vi "Read Status.vi"(8 "error in (no error)":errorcluster, 11 "CSM-Helper in":refnum<class "CSM-Helper.lvclass">) -> (0 "error out":errorcluster, 2 "Array 3":cluster{"Status":string, "InState":string}[](array[cluster]), 3 "CSM-Helper out":refnum<class "CSM-Helper.lvclass">)   [LabVIEW 2017, in "CSM-Helper.lvclass"]
uses:
  CSM-Helper.lvclass
  CSM-Helper.lvclass/CSM-Helper.ctl
  <vilib>/Utility/traverseref.llb/TRef TravTarget.ctl
  <vilib>/Utility/traverseref.llb/VI Scripting - Traverse.lvlib
  Utility/_Support/Terminals.llb/csmHelper-Terminals.lvlib
  _Shared/CSM Shared.lvlib
  Communicable State Machine.lvlib
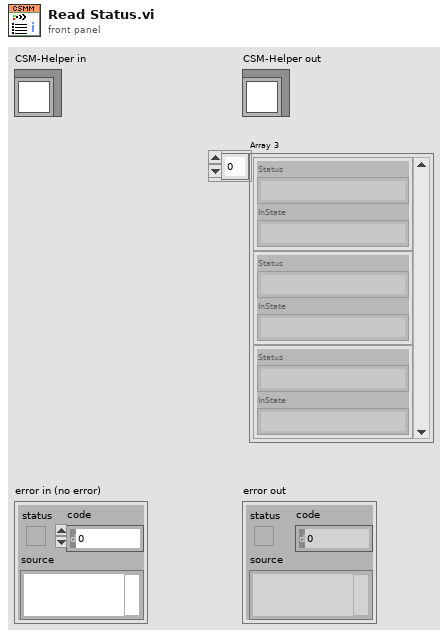
[diagram p1: front panel]
types:
  T1 = typedef "TRef TravTarget.ctl" = enum16{"FP", "BD", "Other"}
  T2 = cluster{"trimed text":string, "trimed text":string}
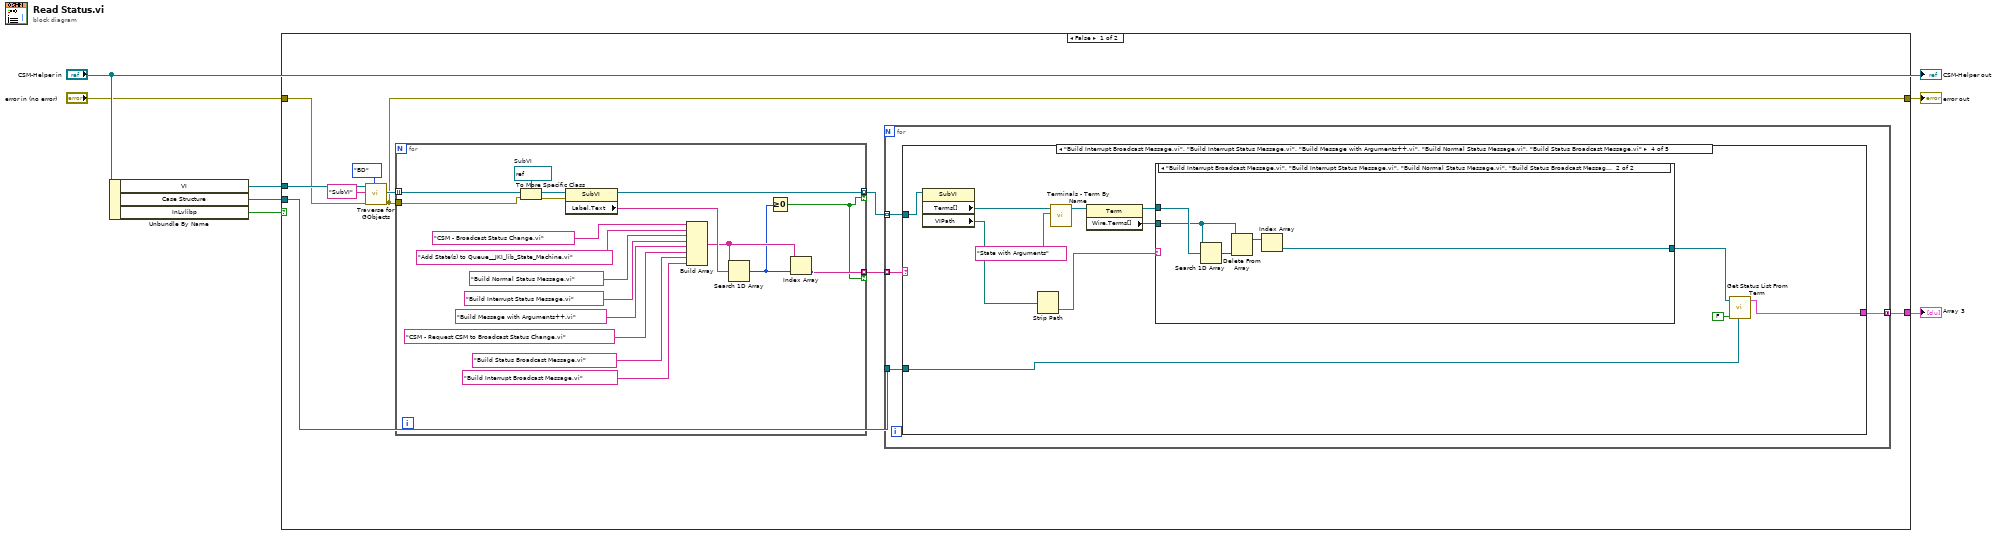
[diagram p0: block diagram]
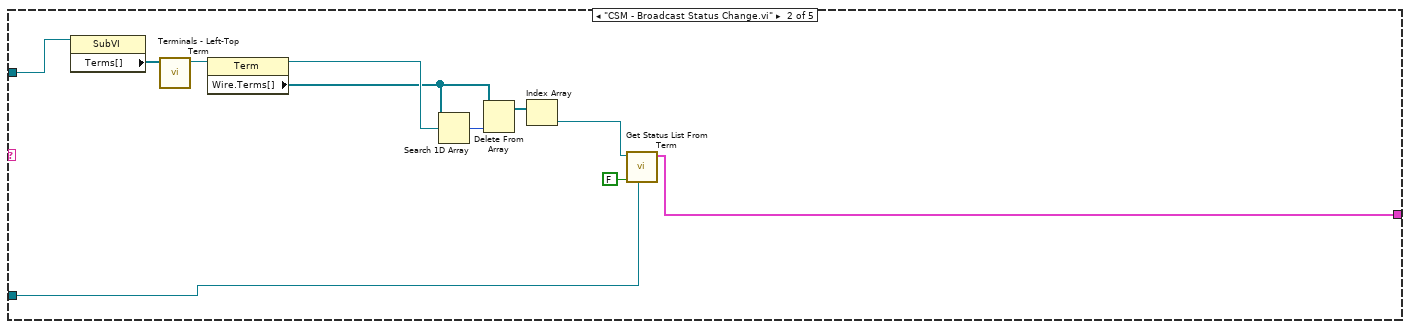
[diagram p3: hidden frame]
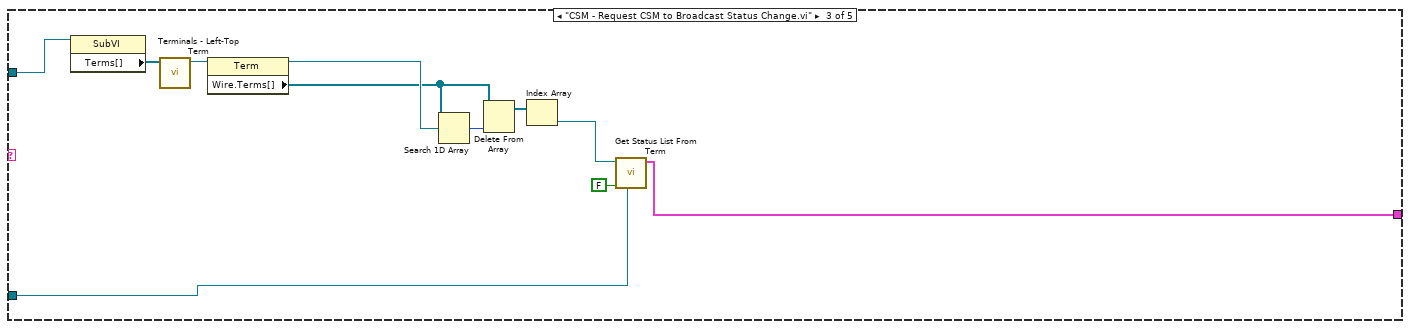
[diagram p4: hidden frame]
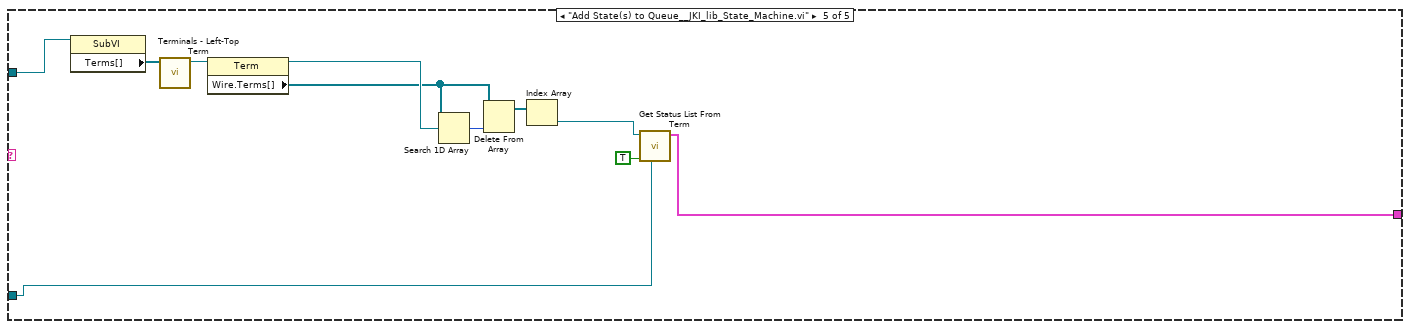
[diagram p6: hidden frame]
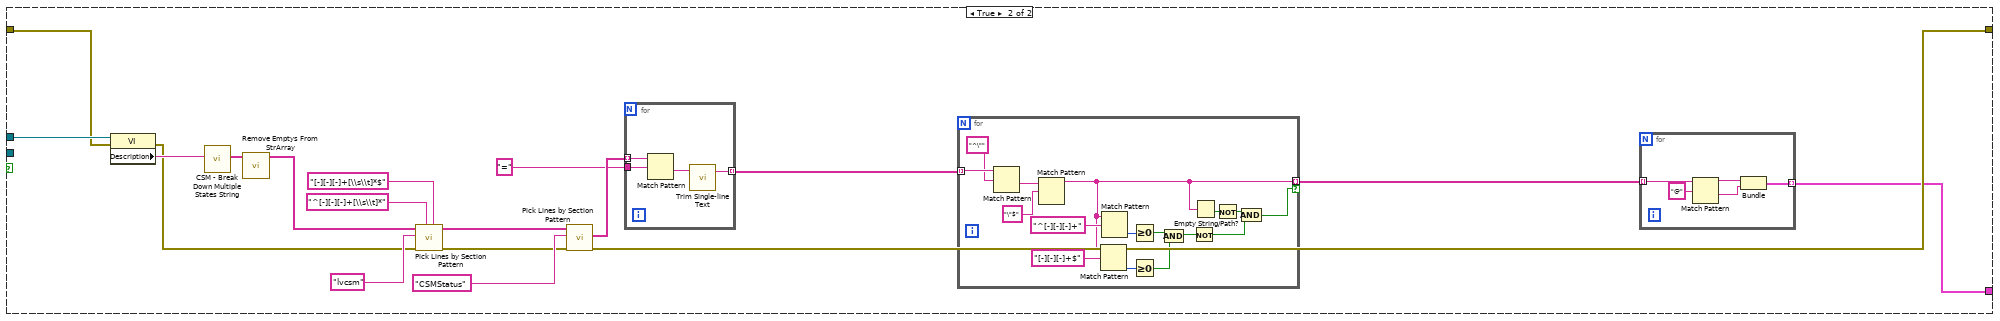
[diagram p7: hidden frame]
diagram:
  n1 = Unbundle By Name("CSM-Helper in") -> ("VI"=w6:refnum<vi>, "Case Structure"=w4:refnum<vi>, "InLvlibp"=w3:bool)
  n2 = case shown="False" w3 {
    tunnel: w6 -> [w13 w96]
    tunnel: [w12 w93] -> w5
    tunnel: w4 -> [w11 _]
    tunnel: "error in (no error)" -> [w9 w95]
    tunnel: [w8 w94] -> w1
    frame False {
      n3 = call <vilib>:"Traverse for GObjects.vi"("Traverse Target"=TRef_TravTarget."BD", "error in (no error)"=w9, "Class Name"="SubVI", "VI Refnum"=w13) -> ("error out"=w8:errorcluster, "References"=w15:refnum<vi>[])  [unwired: 4 in, 2 out]
      n4 = for {
        tunnel: w15 -> [w90] mode=indexing
        tunnel: w8 -> [w86]
        tunnel: [w84] -> w14 mode=indexing if=w78
        tunnel: [w79] -> w10 mode=indexing if=w78
        w87 = refnum<vi> refnum  # SubVI
        n5 = To More Specific Class(target class=w87, reference=w90, error in=w86) -> (specific class reference=w89:refnum<vi>, error out=w88:errorcluster)
        n6 = property class="SubVI"(reference=w89, error in=w88) -> (reference out=w84:refnum<vi>, "Label.Text"=w82:string)  [unwired: 1 out]
        n7 = Build Array("CSM - Broadcast Status Change.vi" ("y"), "Add State(s) to Queue__JKI_lib_State_Machine.vi" ("y"), "Build Normal Status Message.vi" ("y"), "Build Interrupt Status Message.vi" ("y"), "Build Message with Arguments++.vi" ("y"), "CSM - Request CSM to Broadcast Status Change.vi" ("y"), "Build Status Broadcast Message.vi" ("y"), "Build Interrupt Broadcast Message.vi" ("y")) -> (w81:string[])
        n8 = Search 1D Array(1D array=w81, element=w82) -> (index of element=w80:i32)  [unwired: 1 in]
        n9 = Greater Or Equal To 0?(x=w80) -> (x >= 0?=w78:bool)
        n10 = Index Array(array=w81, index=w80) -> (element=w79:string)
      }
      n11 = for {
        tunnel: w14 -> [w21] mode=indexing
        tunnel: [w20] -> w12 mode=concatenating
        tunnel: w11 -> [w19]
        tunnel: w10 -> [w18] mode=indexing
        n12 = case shown="\"Build Interrupt Broadcast Message.vi\", \"Build Interrupt Status Message.vi\", \"Build Message with Arguments++.vi\", \"Build Normal Status Message.vi\", \"Build Status Broadcast Message.vi\"" w18 {
          tunnel: w21 -> [_ w32 w43 w55 w71]
          tunnel: [_ w23 w34 w45 w62] -> w20
          tunnel: w19 -> [_ w24 w35 w47 w63]
          frame Default {
          }
          frame "CSM - Broadcast Status Change.vi" {
            n13 = property class="SubVI"(reference=w32) -> ("Terms[]"=w31:refnum<vi>[])  [unwired: 1 in, 2 out]
            n14 = call "Terminals - Left-Top Term.vi"("Terms[]"=w31) -> ("Terms[] out"=w30:refnum<vi>)  [unwired: 10 in]
            n15 = property class="Term"(reference=w30) -> (reference out=w29:refnum<vi>, "Wire.Terms[]"=w27:refnum<vi>[])  [unwired: 1 in, 1 out]
            n16 = Search 1D Array(1D array=w27, element=w29) -> (index of element=w28:i32)  [unwired: 1 in]
            n17 = Delete From Array(array=w27, index=w28) -> (array with subset deleted=w26:refnum<vi>[])  [unwired: 1 in, 1 out]
            n18 = Index Array(array=w26) -> (element=w25:refnum<vi>)  [unwired: 1 in]
            n19 = call "Get Status List From Term.vi"("CSM CaseRef"=w24, "need Symbol?"=FALSE, "Term Refnum"=w25) -> ("Array"=w23:cluster{"Status":string, "InState":string}[])  [unwired: 6 in]
          }
          frame "CSM - Request CSM to Broadcast Status Change.vi" {
            n20 = property class="SubVI"(reference=w43) -> ("Terms[]"=w42:refnum<vi>[])  [unwired: 1 in, 2 out]
            n21 = call "Terminals - Left-Top Term.vi"("Terms[]"=w42) -> ("Terms[] out"=w41:refnum<vi>)  [unwired: 10 in]
            n22 = property class="Term"(reference=w41) -> (reference out=w40:refnum<vi>, "Wire.Terms[]"=w38:refnum<vi>[])  [unwired: 1 in, 1 out]
            n23 = Search 1D Array(1D array=w38, element=w40) -> (index of element=w39:i32)  [unwired: 1 in]
            n24 = Delete From Array(array=w38, index=w39) -> (array with subset deleted=w37:refnum<vi>[])  [unwired: 1 in, 1 out]
            n25 = Index Array(array=w37) -> (element=w36:refnum<vi>)  [unwired: 1 in]
            n26 = call "Get Status List From Term.vi"("CSM CaseRef"=w35, "need Symbol?"=FALSE, "Term Refnum"=w36) -> ("Array"=w34:cluster{"Status":string, "InState":string}[])  [unwired: 6 in]
          }
          frame "Build Interrupt Broadcast Message.vi", "Build Interrupt Status Message.vi", "Build Message with Arguments++.vi", "Build Normal Status Message.vi", "Build Status Broadcast Message.vi" {
            n27 = property class="SubVI"(reference=w55) -> ("Terms[]"=w52:refnum<vi>[], "VIPath"=w49:path)  [unwired: 1 in, 2 out]
            n28 = Strip Path(path=w49) -> (name=w48:string)  [unwired: 1 out]
            n29 = call "Terminals - Term By Name.vi"("String"="State with Arguments", "Terms[]"=w52) -> ("Terms[] out"=w51:refnum<vi>)  [unwired: 9 in]
            n30 = property class="Term"(reference=w51) -> (reference out=w54:refnum<vi>, "Wire.Terms[]"=w53:refnum<vi>[])  [unwired: 1 in, 1 out]
            n31 = case shown="\"Build Interrupt Broadcast Message.vi\", \"Build Interrupt Status Message.vi\", \"Build Normal Status Message.vi\", \"Build Status Broadcast Message.vi\"" w48 {
              tunnel: w54 -> [_ w60]
              tunnel: w53 -> [_ w58]
              tunnel: [_ w56] -> w46
              frame "False", Default {
              }
              frame "Build Interrupt Broadcast Message.vi", "Build Interrupt Status Message.vi", "Build Normal Status Message.vi", "Build Status Broadcast Message.vi" {
                n32 = Search 1D Array(1D array=w58, element=w60) -> (index of element=w59:i32)  [unwired: 1 in]
                n33 = Delete From Array(array=w58, index=w59) -> (array with subset deleted=w57:refnum<vi>[])  [unwired: 1 in, 1 out]
                n34 = Index Array(array=w57) -> (element=w56:refnum<vi>)  [unwired: 1 in]
              }
            }
            n35 = call "Get Status List From Term.vi"("CSM CaseRef"=w47, "need Symbol?"=FALSE, "Term Refnum"=w46) -> ("Array"=w45:cluster{"Status":string, "InState":string}[])  [unwired: 6 in]
          }
          frame "Add State(s) to Queue__JKI_lib_State_Machine.vi" {
            n36 = property class="SubVI"(reference=w71) -> ("Terms[]"=w70:refnum<vi>[])  [unwired: 1 in, 2 out]
            n37 = call "Terminals - Left-Top Term.vi"("Terms[]"=w70) -> ("Terms[] out"=w69:refnum<vi>)  [unwired: 10 in]
            n38 = property class="Term"(reference=w69) -> (reference out=w68:refnum<vi>, "Wire.Terms[]"=w66:refnum<vi>[])  [unwired: 1 in, 1 out]
            n39 = Search 1D Array(1D array=w66, element=w68) -> (index of element=w67:i32)  [unwired: 1 in]
            n40 = Delete From Array(array=w66, index=w67) -> (array with subset deleted=w65:refnum<vi>[])  [unwired: 1 in, 1 out]
            n41 = Index Array(array=w65) -> (element=w64:refnum<vi>)  [unwired: 1 in]
            n42 = call "Get Status List From Term.vi"("CSM CaseRef"=w63, "need Symbol?"=TRUE, "Term Refnum"=w64) -> ("Array"=w62:cluster{"Status":string, "InState":string}[])  [unwired: 6 in]
          }
        }
      }
    }
    frame True {
      n43 = property class="VI"(reference=w96, error in=w95) -> (error out=w103:errorcluster, "Description"=w104:string)  [unwired: 1 out]
      n44 = call "CSM - Break Down Multiple States String.vi"("States"=w104) -> ("Multiple States"=w98:string[])  [unwired: 10 in]
      n45 = call "Remove Emptys From StrArray.vi"("Array In"=w98) -> ("Array Out"=w97:string[])  [unwired: 10 in]
      n46 = call "Pick Lines by Section Pattern.vi"("RegExp Right(\"^[\")"="[-][-][-]+[\\s\\t]*$" ("RegExp Lef(\"^[\")"), "RegExp Lef(\"^[\")"="^[-][-][-]+[\\s\\t]*" ("RegExp Lef(\"^[\")"), "error in (no error)"=w103, "Session Name"="lvcsm" ("[] Session Name"), "Config Text List"=w97) -> ("error out"=w102:errorcluster, "Config Text List out"=w101:string[])  [unwired: 2 in, 3 out]
      n47 = call "Pick Lines by Section Pattern.vi"("error in (no error)"=w102, "Session Name"="CSMStatus" ("[] Session Name"), "Config Text List"=w101) -> ("error out"=w94:errorcluster, "Session"=w107:string[])  [unwired: 4 in, 3 out]
      n48 = for {
        tunnel: w107 -> [w133] mode=indexing
        tunnel: "=" ("regular expression") -> [w132]
        tunnel: [w130] -> w92 mode=indexing
        n49 = Match Pattern(string=w133, regular expression=w132) -> (after substring=w131:string)  [unwired: 1 in, 3 out]
        n50 = call "Trim Single-line Text.vi"("single-line text"=w131) -> ("trimed text"=w130:string)  [unwired: 2 in]
      }
      n51 = for {
        tunnel: w92 -> [w124] mode=indexing
        tunnel: [w109] -> w91 mode=indexing if=w113
        n52 = Match Pattern(string=w124, regular expression="^\"") -> (after substring=w122:string)  [unwired: 1 in, 3 out]
        n53 = Match Pattern(string=w122, regular expression="\"$") -> (before substring=w109:string)  [unwired: 1 in, 3 out]
        n54 = Match Pattern(string=w109, regular expression="[-][-][-]+$") -> (offset past match=w117:i32)  [unwired: 1 in, 3 out]
        n55 = Match Pattern(string=w109, regular expression="^[-][-][-]+") -> (offset past match=w118:i32)  [unwired: 1 in, 3 out]
        n56 = Greater Or Equal To 0?(x=w118) -> (x >= 0?=w116:bool)
        n57 = Greater Or Equal To 0?(x=w117) -> (x >= 0?=w115:bool)
        n58 = And(x=w116, y=w115) -> (x .and. y?=w114:bool)
        n59 = Not(x=w114) -> (.not. x?=w112:bool)
        n60 = Empty String/Path?(string/path=w109) -> (empty?=w111:bool)
        n61 = Not(x=w111) -> (.not. x?=w110:bool)
        n62 = And(x=w110, y=w112) -> (x .and. y?=w113:bool)
      }
      n63 = for {
        tunnel: w91 -> [w129] mode=indexing
        tunnel: [w125] -> w93 mode=indexing
        n64 = Match Pattern(string=w129, regular expression="@") -> (before substring=w127:string, after substring=w126:string)  [unwired: 1 in, 2 out]
        n65 = Bundle("trimed text"=w127, "trimed text"=w126) -> (w125:T2)  [unwired: 1 in]
      }
    }
  }
  "error out" <- w1
  "Array 3" <- w5
  "CSM-Helper out" <- "CSM-Helper in"
